vi "Gui_Set_Gas_Refs.vi"(8 "error in (no error)":errorcluster, 9 "Path":path, 10 "EXPERIMENT Inputs":T1={"Setup"="", "Date"="", "User Name"="", "Comment"="", "Experiment Procedures"=[], "Chemical Source"="", "Sample Components"=[], "Species"=[], "Laser 1"={"Used"=TRUE, "Name"="Spectroscopy", "Wavelength"=1000.0, "Energy"=25.0}, "Laser 2"={"Used"=TRUE, "Name"="Spectroscopy", "Wavelength"=1000.0, "Energy"=25.0}, "Laser 3"={"Used"=TRUE, "Name"="Spectroscopy", "Wavelength"=1000.0, "Energy"=25.0}, "Laser 4"={"Used"=TRUE, "Name"="Spectroscopy", "Wavelength"=1000.0, "Energy"=25.0}, "Laser 5"={"Used"=TRUE, "Name"="Spectroscopy", "Wavelength"=1000.0, "Energy"=25.0}, "Lamp 1"={"Used"=TRUE, "Name"="Spectroscopy", "Wavelength"=1000.0, "Attenuation"=25.0}, "Lamp 2"={"Used"=TRUE, "Name"="Spectroscopy", "Wavelength"=1000.0, "Attenuation"=25.0}, "Gas 1"={"Used"=TRUE, "Name"="Spectroscopy", "Pressure"=1000.0}, "Gas 2"={"Used"=TRUE, "Name"="Spectroscopy", "Pressure"=1000.0}, "Gas 3"={"Used"=TRUE, "Name"="Spectroscopy", "Pressure"=1000.0}, "Gas 4"={"Used"=TRUE, "Name"="Spectroscopy", "Pressure"=1000.0}, "Gas 5"={"Used"=TRUE, "Name"="Spectroscopy", "Pressure"=1000.0}}, 11 "Gas Refs":refnum<vi>[](array[refnum])) -> (0 "error out":errorcluster caption="sortie d'erreur", 3 "Gas Refs out":refnum<vi>[](array[refnum]))   [LabVIEW 2020]
doc: "This VI fills all the Gas ring lists with values read from a text file.\nA table of references to the Gas cluster controls is used."
uses:
  controls/EXPERIMENT_Inputs.ctl
  controls/LASER_Inputs.ctl
  controls/LAMP_Inputs.ctl
  controls/GAS_Inputs.ctl
panel:
  # "Lasers"
  # "nm"
  # "mJ"
  # "Lamps"
  # "nm"
  # "dB"
  # "Gas"
  # "bar"
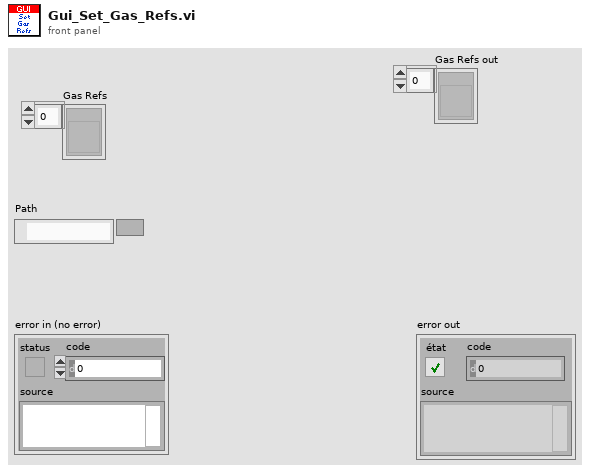
[diagram p1: front panel]
types:
  T1 = typedef "EXPERIMENT_Inputs.ctl" = cluster{"Setup":string, "Date":string, "User Name":string, "Comment":string, "Experiment Procedures":string[], "Chemical Source":string, "Sample Components":string[], "Species":string[], "Laser 1":T2, "Laser 2":T2, "Laser 3":T2, "Laser 4":T2, "Laser 5":T2, "Lamp 1":T3, "Lamp 2":T3, "Gas 1":T4, "Gas 2":T4, "Gas 3":T4, "Gas 4":T4, "Gas 5":T4}
  T2 = typedef "LASER_Inputs.ctl" = cluster{"Used":bool, "Name":string, "Wavelength":dbl, "Energy":dbl}
  T3 = typedef "LAMP_Inputs.ctl" = cluster{"Used":bool, "Name":string, "Wavelength":dbl, "Attenuation":dbl}
  T4 = typedef "GAS_Inputs.ctl" = cluster{"Used":bool, "Name":string, "Pressure":dbl}
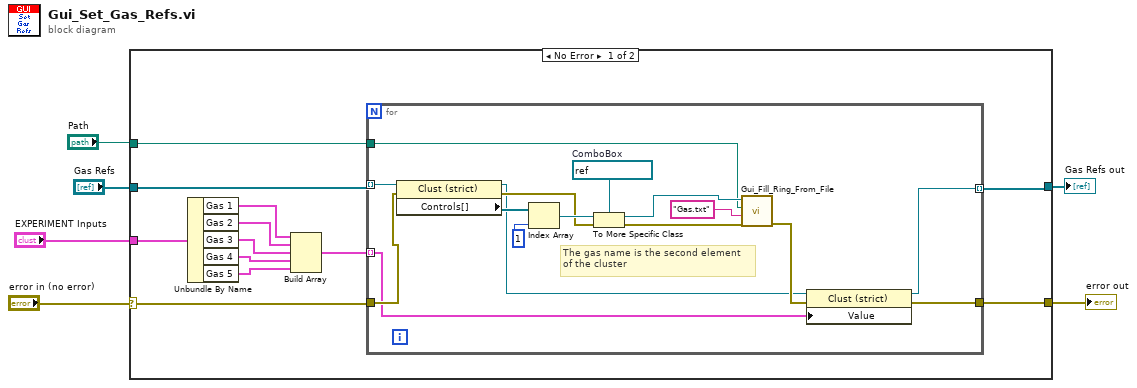
[diagram p0: block diagram]
diagram:
  n1 = case shown="No Error" "error in (no error)" {
    selector: "error in (no error)" -> [w18 w36]
    tunnel: [w9 w36] -> w6
    tunnel: "Gas Refs" -> [w11 w35]
    tunnel: [w10 w35] -> w2
    tunnel: "Path" -> [w8 _]
    tunnel: "EXPERIMENT Inputs" -> [w7 _]
    frame No Error {
      n2 = Unbundle By Name(w7) -> ("Gas 1"=w13:T4, "Gas 2"=w14:T4, "Gas 3"=w15:T4, "Gas 4"=w16:T4, "Gas 5"=w17:T4)
      n3 = Build Array(w13, w14, w15, w16, w17) -> (w12:T4[])
      n4 = for {
        tunnel: w12 -> [w19] mode=indexing
        tunnel: w11 -> [w26] mode=indexing
        tunnel: [w34] -> w10 mode=indexing
        tunnel: w18 -> [w25]
        tunnel: [w33] -> w9
        tunnel: w8 -> [w23]
        w27 = refnum<vi> refnum  # ComboBox
        # "The gas name is the second element\nof the cluster"
        n5 = property class="Clust (strict)"(reference=w26, error in=w25) -> (reference out=w21:refnum<vi>, error out=w24:errorcluster, "Controls[]"=w31:refnum<vi>[])
        n6 = Index Array(array=w31, index=1 ("indice")) -> (element=w29:refnum<vi>)
        n7 = To More Specific Class(target class=w27, reference=w29, error in=w24) -> (specific class reference=w28:refnum<vi>, error out=w20:errorcluster)
        n8 = call "Gui_Fill_Ring_From_File.vi"("error in (no error)"=w20, "Resource Name"="Gas.txt", "Resource Path"=w23, "Refnum ChneDér"=w28) -> ("error out"=w22:errorcluster)  [unwired: 4 in, 3 out]
        n9 = property class="Clust (strict)"(reference=w21, error in=w22, "Value"=w19) -> (reference out=w34:refnum<vi>, error out=w33:errorcluster)
      }
    }
    frame Error {
    }
  }
  "error out" <- w6
  "Gas Refs out" <- w2
